vi "Global - Comport.vi"() -> ()   [LabVIEW 2019]
panel:
  in  "Port":string[](array[string])
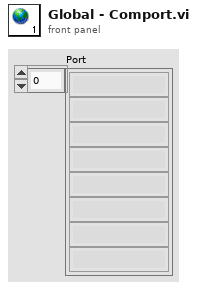
[diagram p1: front panel]
diagram:
